vi "acquire_in_tag_lens_direction.vi"(2 "iterations until end of fly-back scan segment":u16, 3 "iterations until start of fly-back scan segment":u16, 4 "iterations per scan segment":u16, 5 "iteration counter (resonance cycle) out":u16) -> (0 "flyback phase?":bool, 1 "acquire during flyforward or flyback phase?":bool)   [LabVIEW 2010]
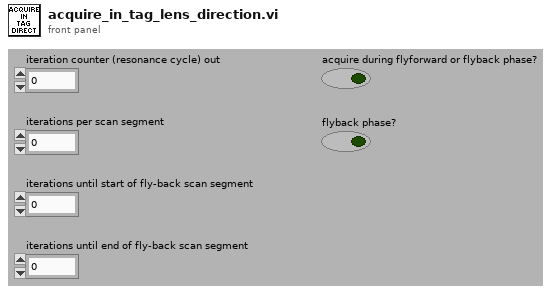
[diagram p1: front panel]
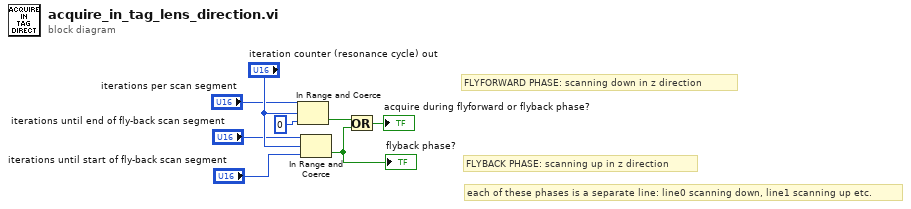
[diagram p0: block diagram]
diagram:
  # "each of these phases is a separate line: line0 scanning down, line1 scanning up etc."
  # "FLYBACK PHASE: scanning up in z direction"
  # "FLYFORWARD PHASE: scanning down in z direction"
  n1 = In Range and Coerce(upper limit="iterations per scan segment", x="iteration counter (resonance cycle) out", lower limit=u16 0) -> (In Range?=w3:bool)  [unwired: 1 out]
  n2 = In Range and Coerce(upper limit="iterations until end of fly-back scan segment", x="iteration counter (resonance cycle) out", lower limit="iterations until start of fly-back scan segment") -> (In Range?=w7:bool)  [unwired: 1 out]
  "flyback phase?" <- w7
  n3 = Or(x=w3, y=w7) -> (x .or. y?=→"acquire during flyforward or flyback phase?":bool)
